vi "setTriggerIn.vi"(0 "CCD in":refnum<class "CCD.lvclass">, 1 "enable":bool=TRUE, 5 "address":i32, 7 "event":i32, 9 "signalType":i32, 11 "error in (no error)":errorcluster, 12 "Delay between send and receive [ms]":i32=100) -> (4 "CCD out":refnum<class "CCD.lvclass">, 6 "results-JSON string":string, 8 "ID":i32, 15 "error out":errorcluster)   [LabVIEW 2023, in "CCD.lvclass"]
uses:
  CCD.lvclass
  CCD.lvclass/CCD.ctl
  20f7d3bd-08ac-4524-9bed-df36c1da25a0.vi
  GenericDevice/GenericDevice.lvclass
  cab240a6-cbf4-4e2c-ab79-96d9c1b88265.vi
  <vilib>/IlluminatedG/lv-web-crypto/lv-json/JSON/JSON.lvlib
  836cf838-2038-4e61-ba77-441fbdd5e01c.vi
  46ee8d0c-dc08-4fbc-92d1-4c6f5c678b17.vi
  ef38dbf6-39c5-45e7-8746-a7131d194a3a.vi
panel:
  # "Connector Pane"
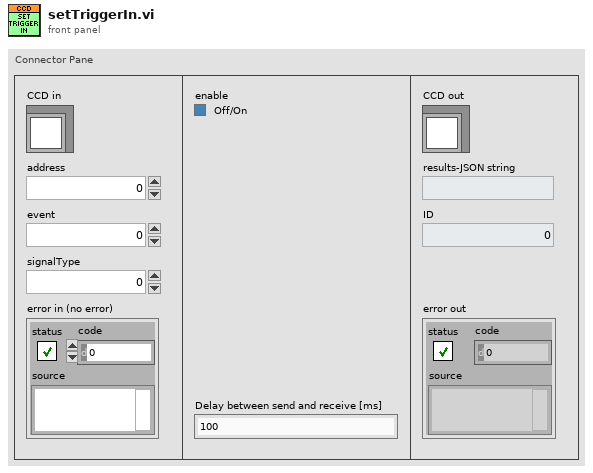
[diagram p1: front panel]
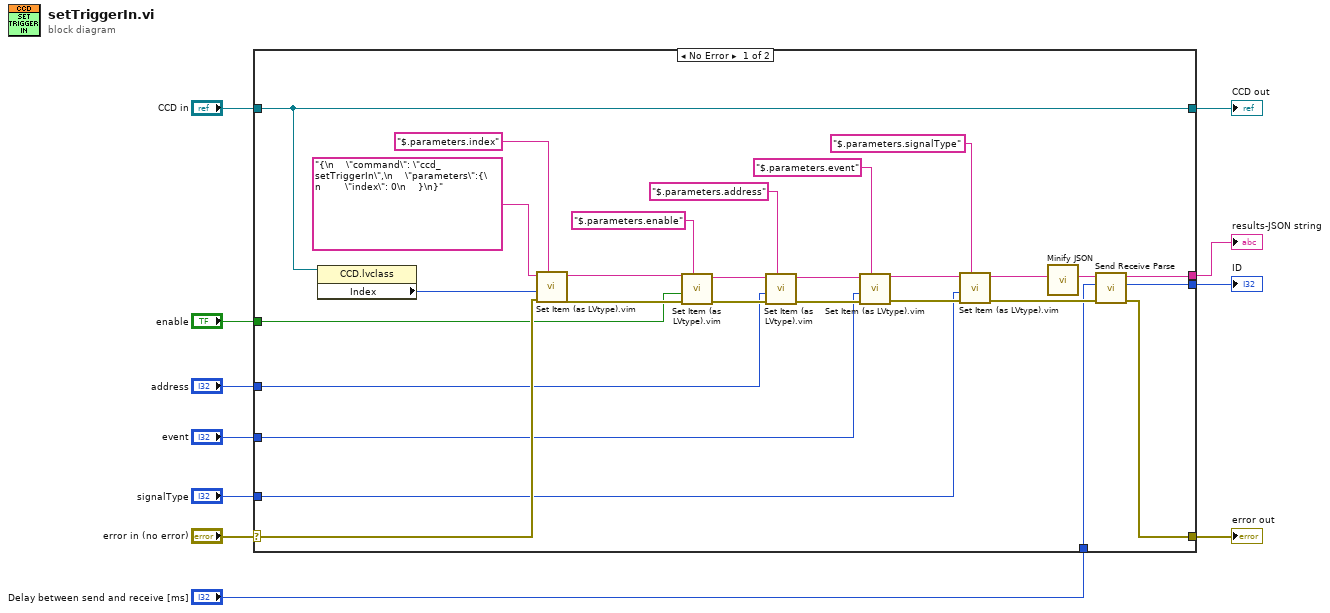
[diagram p0: block diagram]
diagram:
  n1 = case shown="No Error" "error in (no error)" {
    selector: "error in (no error)" -> [w35 w41]
    tunnel: [w31 w41] -> w10
    tunnel: [w37 w40] -> w8
    tunnel: "CCD in" -> [w37 w40]
    tunnel: [w30 _] -> w7
    tunnel: [w29 _] -> w1
    tunnel: "enable" -> [w27 _]
    tunnel: "Delay between send and receive [ms]" -> [w15 _]
    tunnel: "address" -> [w14 _]
    tunnel: "event" -> [w13 _]
    tunnel: "signalType" -> [w12 _]
    frame No Error {
      n2 = property class="CCD.lvclass"(reference=w37) -> ("Index"=w36:i32)  [unwired: 1 in, 2 out]
      n3 = call "Set Item (as LVtype).vim"("$Path or Item Name"="$.parameters.index", "error in (no error)"=w35, "Anything"=w36, "JSON"="{\n    \"command\": \"ccd_setTriggerIn\",\n    \"parameters\":{\n        \"index\": 0\n    }\n}") -> ("error out"=w33:errorcluster, "<JSON>"=w32:string)  [unwired: 4 in, 1 out]
      n4 = call "Set Item (as LVtype).vim"("$Path or Item Name"="$.parameters.enable", "error in (no error)"=w33, "Anything"=w27, "JSON"=w32) -> ("error out"=w23:errorcluster, "<JSON>"=w19:string)  [unwired: 4 in, 1 out]
      n5 = call "Set Item (as LVtype).vim"("$Path or Item Name"="$.parameters.address", "error in (no error)"=w23, "Anything"=w14, "JSON"=w19) -> ("error out"=w20:errorcluster, "<JSON>"=w16:string)  [unwired: 4 in, 1 out]
      n6 = call "Set Item (as LVtype).vim"("$Path or Item Name"="$.parameters.event", "error in (no error)"=w20, "Anything"=w13, "JSON"=w16) -> ("error out"=w21:errorcluster, "<JSON>"=w17:string)  [unwired: 4 in, 1 out]
      n7 = call "Set Item (as LVtype).vim"("$Path or Item Name"="$.parameters.signalType", "error in (no error)"=w21, "Anything"=w12, "JSON"=w17) -> ("error out"=w22:errorcluster, "<JSON>"=w18:string)  [unwired: 4 in, 1 out]
      n8 = call <vilib>:"Minify JSON.vi"("JSON String"=w18) -> ("Minified JSON"=w28:string)  [unwired: 10 in]
      n9 = call "Send Receive Parse.vi"("error in"=w22, "Delay between send and receive [ms]"=w15, "<JSON>"=w28) -> ("error out"=w31:errorcluster, "ID"=w29:i32, "results-JSON string"=w30:string)  [unwired: 6 in]
    }
    frame Error {
    }
  }
  "error out" <- w10
  "CCD out" <- w8
  "results-JSON string" <- w7
  "ID" <- w1
